vi "Security System.vi"() -> ()   [LabVIEW 2013]
doc: "This VI simulates the security system by monitoring the alarm switches, bypass switches, tamper switches and indicates the corresponding activity with different colours."
uses:
  Controls/Security System Indicators.ctl
  Controls/Security System States.ctl
  Controls/Log File States.ctl
panel:
  in  "stop simulation":bool
  out "Zone status indicators":T1
  in  "Tamper switches":bool[](array[boolean])
  in  "Bypass Switches":bool[](array[boolean])
  in  "Alarm Switches":bool[](array[boolean])
  # "· Green: Normal\n· Red: Alarm\n· Blue: Bypass\n· Orange: Tampe"
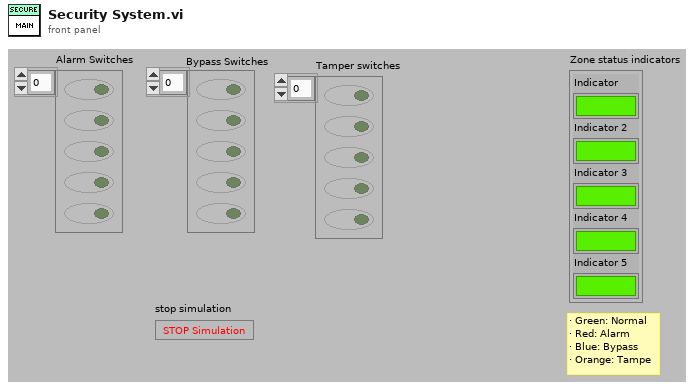
[diagram p1: front panel]
types:
  T1 = typedef "Security System Indicators.ctl" = cluster{"Indicator":bool, "Indicator 2":bool, "Indicator 3":bool, "Indicator 4":bool, "Indicator 5":bool}
  T2 = typedef "Security System States.ctl" = enum16{"Initialize", "Main", "Process", "Stop"}
  T3 = typedef "Log File States.ctl" = enum16{"Initialize", "Write", "Stop"}
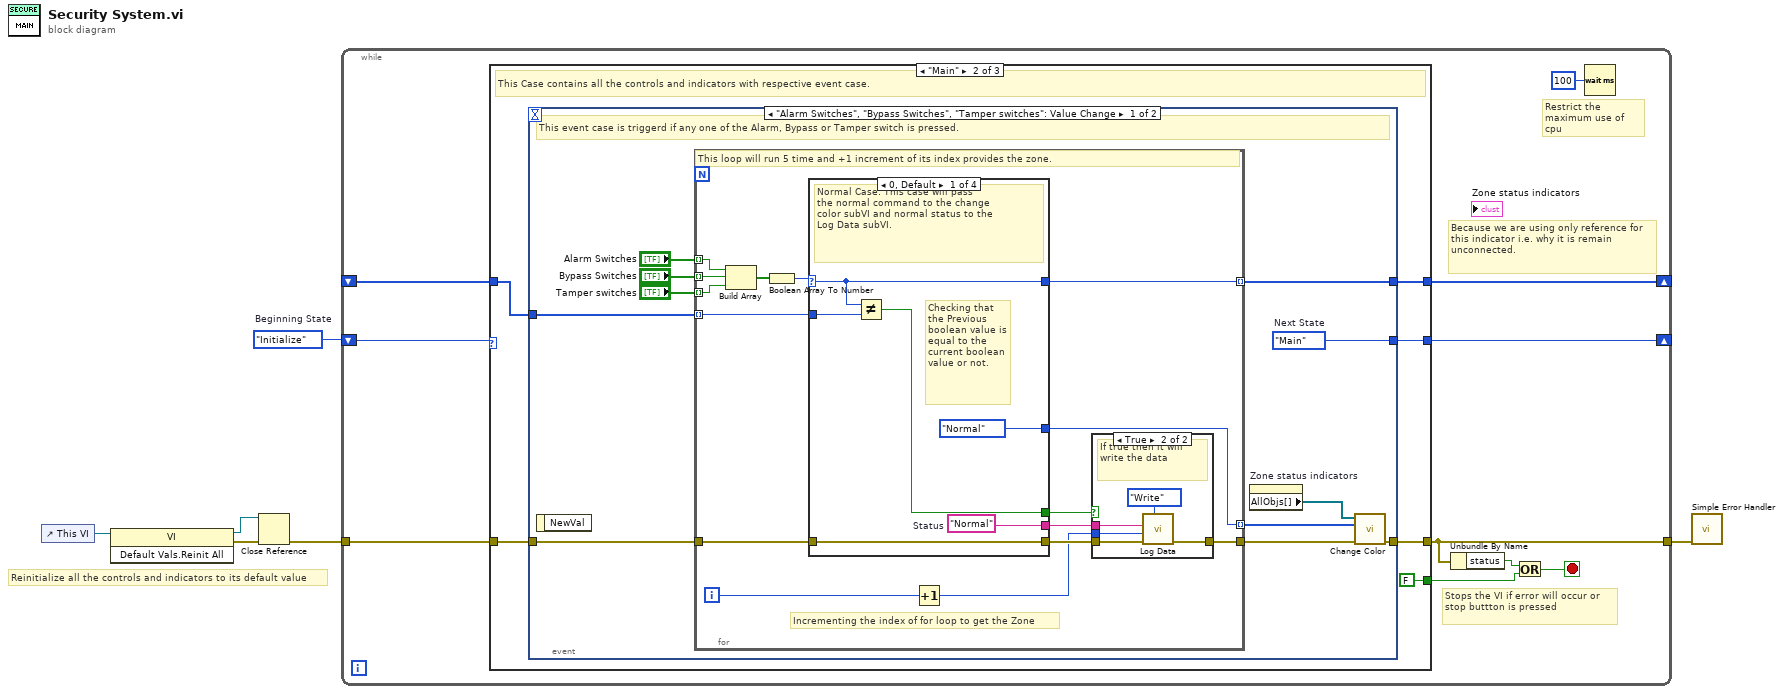
[diagram p0: block diagram]
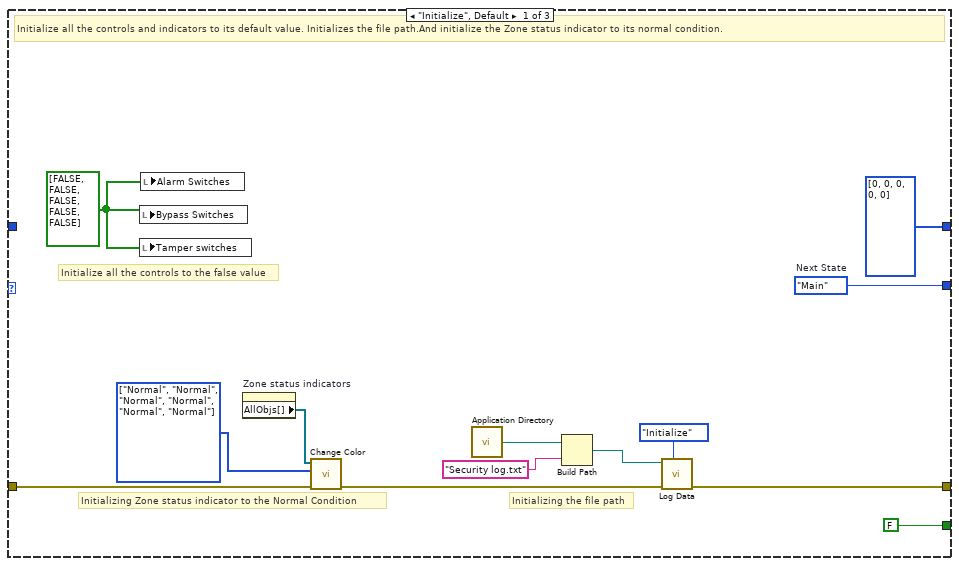
[diagram p2: hidden frame]
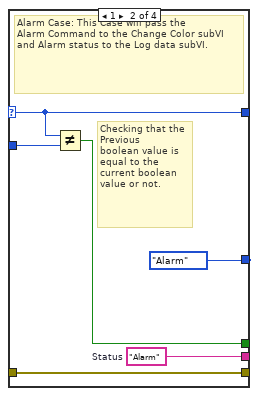
[diagram p4: hidden frame]
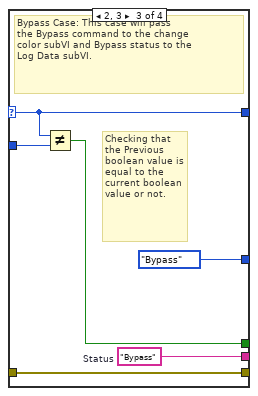
[diagram p5: hidden frame]
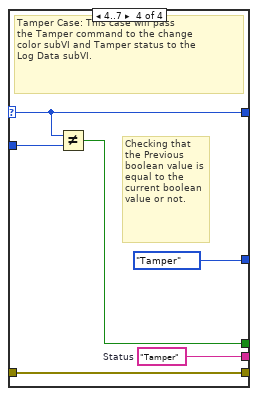
[diagram p6: hidden frame]
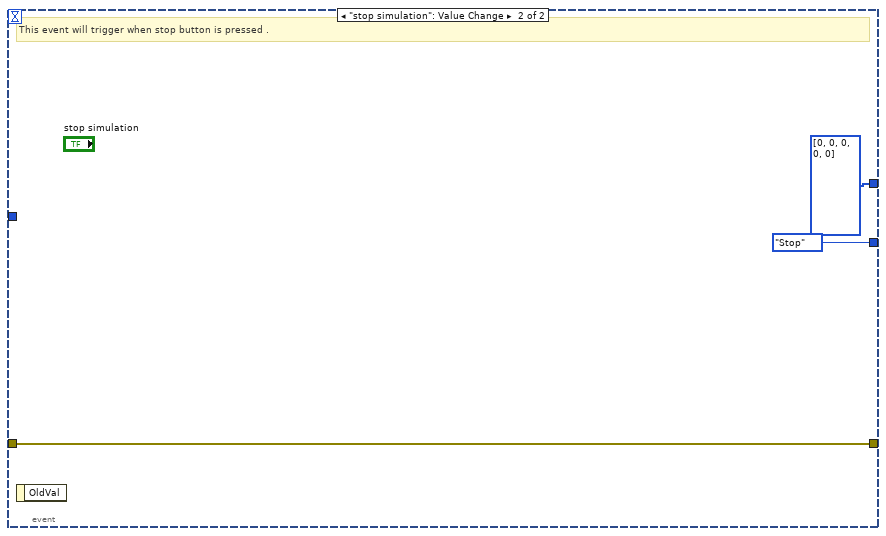
[diagram p7: hidden frame]
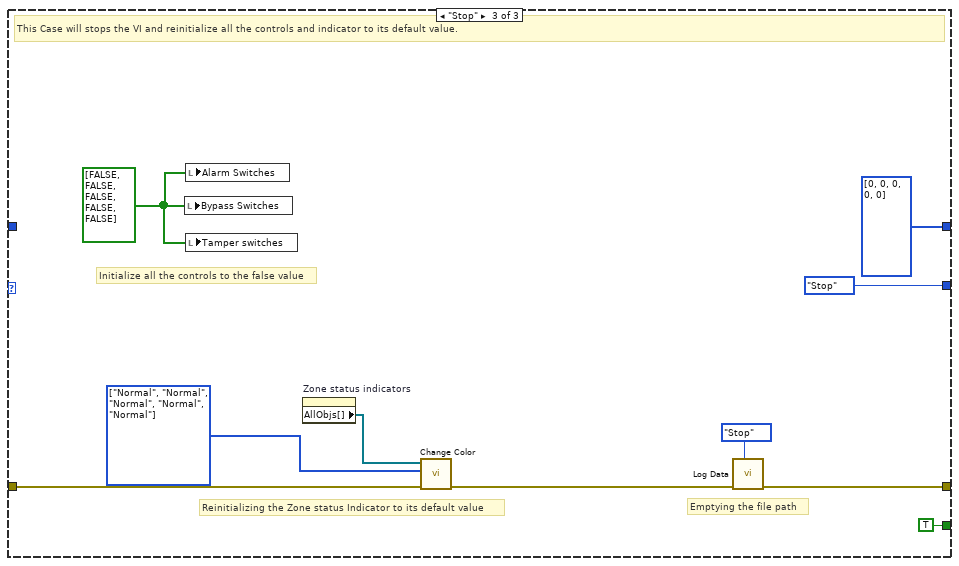
[diagram p8: hidden frame]
diagram:
  w6 = Security_System_States."Initialize"  # Beginning State
  # "Reinitialize all the controls and indicators to its default value"
  n1 = control-ref of="This VI"() -> (w5:refnum<vi>)
  n2 = invoke class="VI" method="Default Vals.Reinit All"(reference=w5) -> (reference out=w3:refnum<vi>, error out=w4:errorcluster)  [unwired: 2 in, 1 out]
  n3 = Close Reference(reference=w3, error in (no error)=w4) -> (error out=w2:errorcluster)
  n4 = while {
    shift-right: [w15] -> _
    shift-left: w6 -> [w16]
    tunnel: [w12] -> w1
    tunnel: w2 -> [w13]
    shift-right: [w8] -> _
    shift-left: _ -> [w7]
    stop <- w9 stop-if-true
    # "Because we are using only reference for this indicator i.e. why it is remain unconnected."
    # "Stops the VI if error will occur or stop buttton is pressed"
    # "Restrict the maximum use of cpu"
    n5 = case shown="\"Main\"" w16 {
      tunnel: [w29 w32 Security_System_States."Stop" ("Next State")] -> w15
      tunnel: [w22 w35 w98] -> w12
      tunnel: w13 -> [w27 w34 w102]
      tunnel: [FALSE FALSE TRUE] -> w10
      tunnel: [u32[] [0, 0, 0, 0, 0] w31 u32[] [0, 0, 0, 0, 0]] -> w8
      tunnel: w7 -> [_ w30 _]
      frame "Initialize", Default {
        w25 = bool[] [FALSE, FALSE, FALSE, FALSE, FALSE] ("Alarm Switches")
        w24 = enum16{"Normal", "Alarm", "Bypass", "Tamper"}[] [enum."Normal", enum."Normal", enum."Normal", enum."Normal", enum."Normal", enum."Normal"] items=["Normal", "Alarm", "Bypass", "Tamper"] ("Command")
        w29 = Security_System_States."Main"  # Next State
        # "Initializing the file path"
        # "Initializing Zone status indicator to the Normal Condition"
        # "Initialize all the controls to the false value"
        # "Initialize all the controls and indicators to its default value. Initializes the file path.And initialize the Zone status indicator to its normal condition."
        n6 = local write "Bypass Switches"(w25) -> ()
        n7 = local write "Tamper switches"(w25) -> ()
        n8 = local write "Alarm Switches"(w25) -> ()
        n9 = property on="Zone status indicators" class="Clust (strict)"() -> ("AllObjs[]"=w26:refnum<vi>[])  [unwired: 2 in, 2 out]
        n10 = call "Change Color.vi"("error in (no error)"=w27, "Command"=w24, "AllObjs[]"=w26) -> ("error out"=w23:errorcluster)  [unwired: 8 in]
        n11 = call <vilib>:"Application Directory.vi"() -> ("Application Directory"=w20:path)
        n12 = Build Path(base path=w20, name or relative path="Security log.txt") -> (appended path=w18:path)
        n13 = call "Log Data.vi"("Command"=Log_File_States."Initialize", "error in (no error)"=w23, "file path"=w18) -> ("error out"=w22:errorcluster)  [unwired: 8 in]
      }
      frame "Main" {
        # "This Case contains all the controls and indicators with respective event case."
        n14 = event shown="[0] \"Alarm Switches\", \"Bypass Switches\", \"Tamper switches\": Value Change" {
          selector: _ -> [_ _]
          dyn-events: _ -> [_ _]
          timeout: _ -> [_ _]
          tunnel: [w40 w93] -> w35
          tunnel: w34 -> [w42 w93]
          tunnel: [w46 Security_System_States."Stop" ("Next State")] -> w32
          tunnel: [w37 u32[] [0, 0, 0, 0, 0]] -> w31
          tunnel: w30 -> [w36 _]
          event "Alarm Switches", "Bypass Switches", "Tamper switches": Value Change {
            w46 = Security_System_States."Main"  # Next State
            # "This event case is triggerd if any one of the Alarm, Bypass or Tamper switch is pressed."
            n15 = event-data() -> ()  [unwired: 1 in, 1 out]
            n16 = for {
              tunnel: "Alarm Switches" -> [w60] mode=indexing
              tunnel: "Bypass Switches" -> [w61] mode=indexing
              tunnel: "Tamper switches" -> [w59] mode=indexing
              tunnel: w42 -> [w57]
              tunnel: [w53] -> w41
              tunnel: [w55] -> w38 mode=indexing
              tunnel: [w50] -> w37 mode=indexing
              tunnel: w36 -> [w49] mode=indexing
              i -> [w51]
              # "Incrementing the index of for loop to get the Zone"
              # "This loop will run 5 time and +1 increment of its index provides the zone."
              n17 = Build Array "Build Array"(w60, w61, w59) -> (w58:bool[])
              n18 = Boolean Array To Number(Boolean array=w58) -> (number=w56:u32)
              n19 = case shown="0, Default" w56 {
                selector: w56 -> [w70 w76 w81 w88]
                tunnel: w57 -> [w73 w79 w85 w91]
                tunnel: [w73 w79 w85 w91] -> w54
                tunnel: [enum16{"Normal", "Alarm", "Bypass", "Tamper"}."Normal" enum16{"Normal", "Alarm", "Bypass", "Tamper"}."Alarm" enum16{"Normal", "Alarm", "Bypass", "Tamper"}."Bypass" enum16{"Normal", "Alarm", "Bypass", "Tamper"}."Tamper"] -> w55
                tunnel: [w71 w77 w83 w89] -> w52
                tunnel: [w70 w76 w81 w88] -> w50
                tunnel: w49 -> [w69 w75 w82 w87]
                tunnel: [w68 w74 w80 w86] -> w48
                frame 0, Default {
                  w71 = "Normal"  # Status
                  # "Checking that the Previous \nboolean value is equal to the \ncurrent boolean value or not."
                  # "Normal Case: This case will pass\nthe normal command to the change\ncolor subVI and normal status to the \nLog Data subVI."
                  n20 = Not Equal?(x=w70, y=w69) -> (x != y?=w68:bool)
                }
                frame 1 {
                  w77 = "Alarm"  # Status
                  # "Checking that the Previous \nboolean value is equal to the \ncurrent boolean value or not."
                  # "Alarm Case: This Case will pass the \nAlarm Command to the Change Color subVI and Alarm status to the Log data subVI."
                  n21 = Not Equal?(x=w76, y=w75) -> (x != y?=w74:bool)
                }
                frame 2, 3 {
                  w83 = "Bypass"  # Status
                  # "Checking that the Previous \nboolean value is equal to the \ncurrent boolean value or not."
                  # "Bypass Case: This case will pass\nthe Bypass command to the change\ncolor subVI and Bypass status to the \nLog Data subVI."
                  n22 = Not Equal?(x=w81, y=w82) -> (x != y?=w80:bool)
                }
                frame 4..7 {
                  w89 = "Tamper"  # Status
                  # "Checking that the Previous \nboolean value is equal to the \ncurrent boolean value or not."
                  # "Tamper Case: This case will pass\nthe Tamper command to the change\ncolor subVI and Tamper status to the \nLog Data subVI."
                  n23 = Not Equal?(x=w88, y=w87) -> (x != y?=w86:bool)
                }
              }
              n24 = Increment(x=w51) -> (x+1=w47:i32)
              n25 = case shown="True" w48 {
                tunnel: w54 -> [w62 w67]
                tunnel: [w62 w66] -> w53
                tunnel: w52 -> [_ w64]
                tunnel: w47 -> [_ w63]
                frame False {
                  # "No action will takes place"
                }
                frame True {
                  # "If true then it will \nwrite the data"
                  n26 = call "Log Data.vi"("Command"=Log_File_States."Write", "error in (no error)"=w67, "Zone"=w63, "Status"=w64) -> ("error out"=w66:errorcluster)  [unwired: 7 in]
                }
              }
            }
            n27 = property on="Zone status indicators" class="Clust (strict)"() -> ("AllObjs[]"=w39:refnum<vi>[])  [unwired: 2 in, 2 out]
            n28 = call "Change Color.vi"("error in (no error)"=w41, "Command"=w38, "AllObjs[]"=w39) -> ("error out"=w40:errorcluster)  [unwired: 8 in]
          }
          event "stop simulation": Value Change {
            # "This event will trigger when stop button is pressed ."
            n29 = event-data() -> ()  [unwired: 1 in, 1 out]
          }
        }
      }
      frame "Stop" {
        w96 = bool[] [FALSE, FALSE, FALSE, FALSE, FALSE] ("Bypass Switches")
        w100 = enum16{"Normal", "Alarm", "Bypass", "Tamper"}[] [enum."Normal", enum."Normal", enum."Normal", enum."Normal", enum."Normal"] items=["Normal", "Alarm", "Bypass", "Tamper"] ("Array")
        # "Initialize all the controls to the false value"
        # "Reinitializing the Zone status Indicator to its default value"
        # "Emptying the file path"
        # "This Case will stops the VI and reinitialize all the controls and indicator to its default value."
        n30 = local write "Bypass Switches"(w96) -> ()
        n31 = local write "Alarm Switches"(w96) -> ()
        n32 = local write "Tamper switches"(w96) -> ()
        n33 = property on="Zone status indicators" class="Clust (strict)"() -> ("AllObjs[]"=w101:refnum<vi>[])  [unwired: 2 in, 2 out]
        n34 = call "Change Color.vi"("error in (no error)"=w102, "Command"=w100, "AllObjs[]"=w101) -> ("error out"=w99:errorcluster)  [unwired: 8 in]
        n35 = call "Log Data.vi"("Command"=Log_File_States."Stop", "error in (no error)"=w99) -> ("error out"=w98:errorcluster)  [unwired: 9 in]
      }
    }
    n36 = Unbundle By Name(w12) -> ("status"=w11:bool)
    n37 = Or(x=w11, y=w10) -> (x .or. y?=w9:bool)
    n38 = Wait (ms)(milliseconds to wait=u32 100) -> ()  [unwired: 1 out]
  }
  n39 = call <vilib>:"Simple Error Handler.vi"("error in (no error)"=w1) -> ()  [unwired: 4 in, 5 out]
